vi "nanomsg_getsocketopt_int.vi"(3 "error in":errorcluster, 4 "option":i32=3, 5 "level":i32=3, 6 "socket in":refnum<class "nanomsg_socket.lvclass">) -> (0 "error out":errorcluster, 1 "value":i32, 2 "socket out":refnum<class "nanomsg_socket.lvclass">)   [LabVIEW 2014, in "nanomsg.lvlib" / "nanomsg_socket.lvclass"]
doc: "Query the value of <b>option</b> for the given <b>socket</b>.\n\nYou are responsible for selecting the correct polymorphic instance for the option you wish to query. Most options return int32; check the API docs or code diagram."
uses:
  nanomsg_socket.lvclass
  nanomsg_socket.lvclass/nanomsg_socket.ctl
  <vilib>/Utility/error.llb/Error Cluster From Error Code.vi
  nanomsg.lvlib
panel:
  # "NN"
  # "labview"
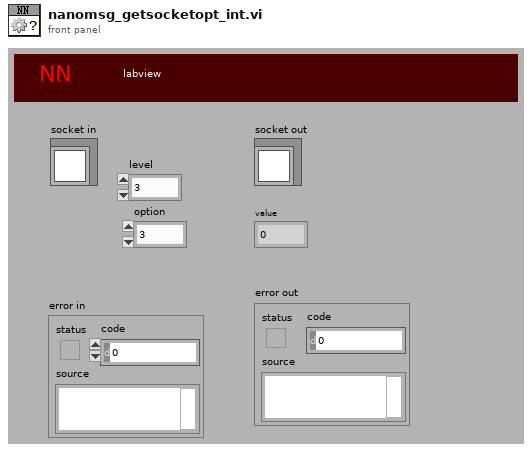
[diagram p1: front panel]
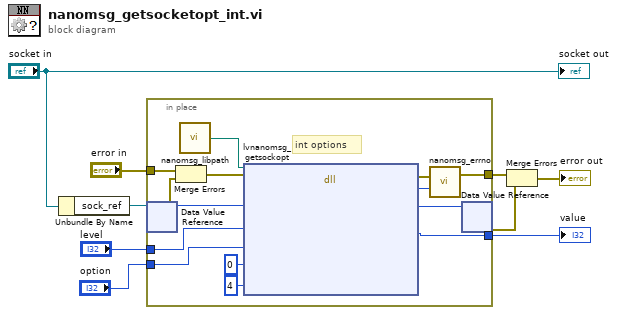
[diagram p0: block diagram]
diagram:
  n1 = Unbundle By Name("socket in") -> ("sock_ref"=w4:refnum<data-value>)
  n2 = in-place {
    in-place-border: [w21] -> w9
    in-place-border: "error in" -> [w20]
    in-place-border: "option" -> [w19]
    in-place-border: [w18] -> w6
    in-place-border: "level" -> [w12]
    # "int options"
    n3 = in-place-dvr #1(w4) -> (w17:u64, w13:errorcluster)
    n4 = Merge Errors(w20, w13) -> (w14:errorcluster)
    n5 = call "nanomsg_libpath.vi"() -> ("path"=w15:path)
    n6 = dll-call lib="?" fn="lvnanomsg_getsockopt" ("zmq_labview.dll:lvzmq_getsockopt")(path in=w15, error in=w14, "socket"=w17, "level"=w12, "option"=w19, "data"=0, "len"=u32 4) -> (error out=w23:errorcluster, "return type"=w22:i32, "socket"=w16:u64, "data"=w18:i32)  [unwired: 4 in, 1 out]
    n7 = call "nanomsg_errno.vi"("retval"=w22, "error in"=w23) -> ("error out"=w21:errorcluster)  [unwired: 1 out]
    n8 = in-place-dvr #1(w16) -> (w2:errorcluster)  [unwired: 1 out]
  }
  "value" <- w6
  n9 = Merge Errors(w9, w2) -> (→"error out":errorcluster)
  "socket out" <- "socket in"
